vi "Parse VTG Sentence.vi"(8 "error in (no error)":errorcluster, 11 "VTG sentence":string) -> (0 "error out":errorcluster, 3 "VTG  data":T1 {"type of fix"."mode" items=["", "Simulator", "Not Valid", "Estimated", "Differential", "Autonomous"]})   [LabVIEW 2011, in "u-blox 5 Series.lvlib"]
doc: "Returns data contained in an NMEA sentence. You must manually select the polymorphic instance to use."
uses:
  u-blox 5 Series.lvlib
  typedefs/VTG Data.ctl
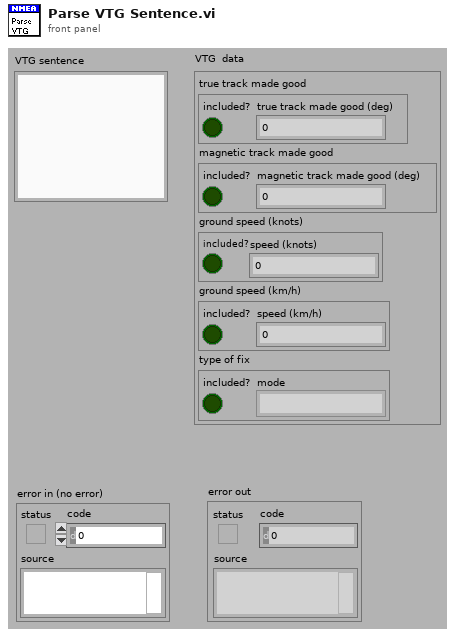
[diagram p1: front panel]
types:
  T1 = typedef "u-blox 5 Series.lvlib/VTG Data.ctl" = cluster{"true track made good":cluster{"included?":bool, "true track made good (deg)":dbl}, "magnetic track made good":cluster{"included?":bool, "magnetic track made good (deg)":dbl}, "ground speed (knots)":cluster{"included?":bool, "speed (knots)":dbl}, "ground speed (km/h)":cluster{"included?":bool, "speed (km/h)":dbl}, "type of fix":cluster{"included?":bool, "mode":u16}}
  T2 = cluster{"Boolean":bool, "True Track Made Good (Deg)":dbl}
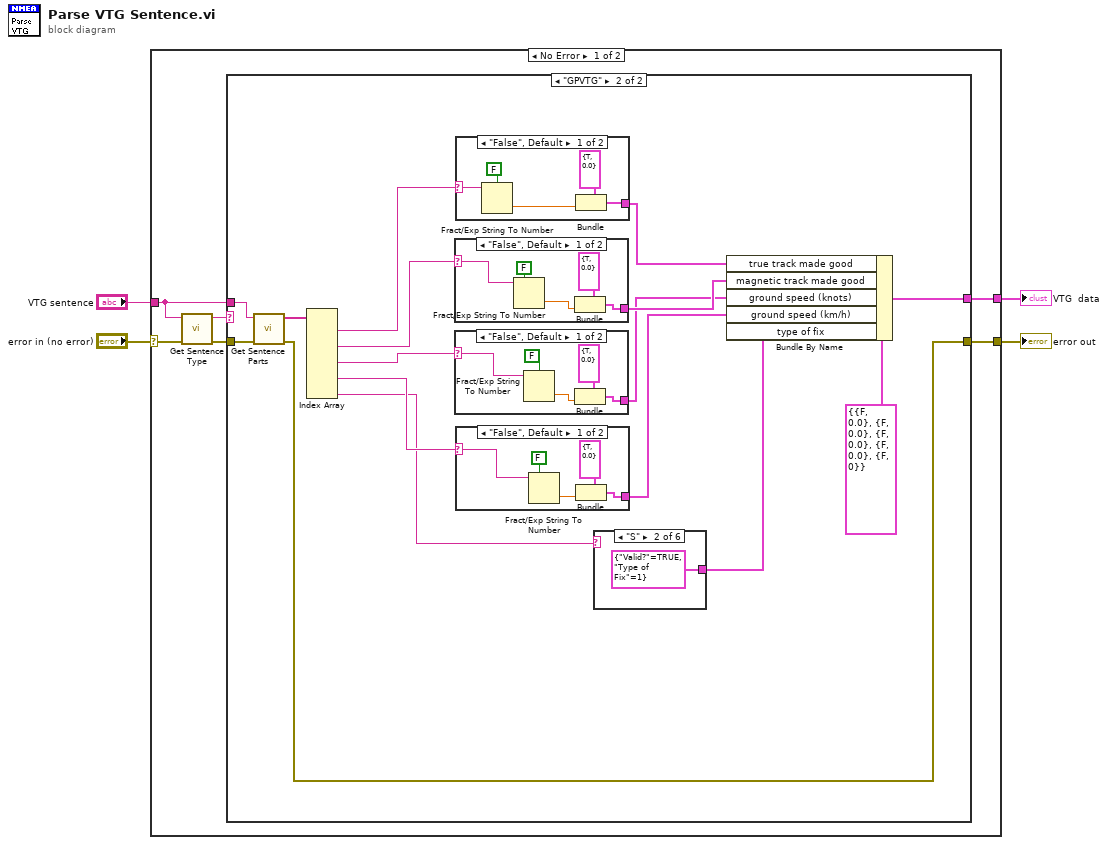
[diagram p0: block diagram]
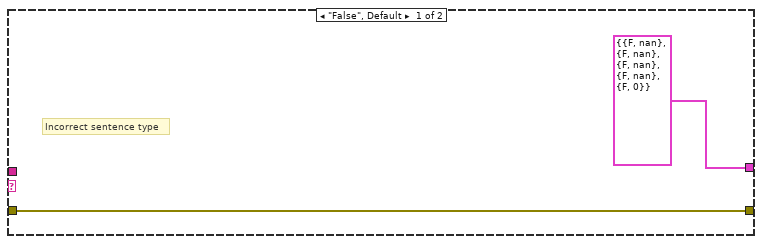
[diagram p2: hidden frame]
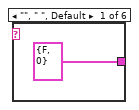
[diagram p3: hidden frame]
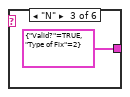
[diagram p4: hidden frame]
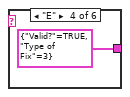
[diagram p5: hidden frame]
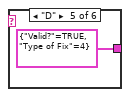
[diagram p6: hidden frame]
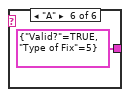
[diagram p7: hidden frame]
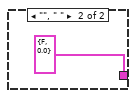
[diagram p8: hidden frame]
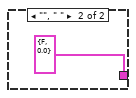
[diagram p9: hidden frame]
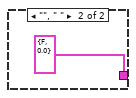
[diagram p10: hidden frame]
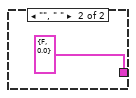
[diagram p11: hidden frame]
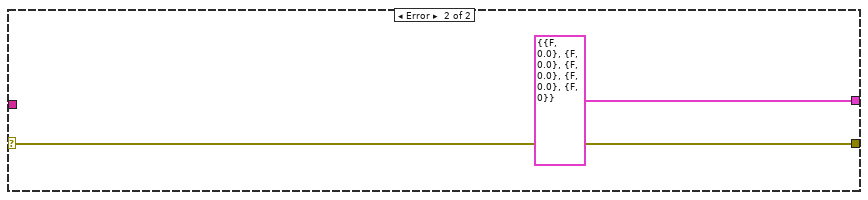
[diagram p12: hidden frame]
diagram:
  n1 = case shown="No Error" "error in (no error)" {
    selector: "error in (no error)" -> [w8 w59]
    tunnel: [w10 T1 {"true track made good"={"included?"=FALSE, "true track made good (deg)"=0.0}, "magnetic track made good"={"included?"=FALSE, "magnetic track made good (deg)"=0.0}, "ground speed (knots)"={"included?"=FALSE, "speed (knots)"=0.0}, "ground speed (km/h)"={"included?"=FALSE, "speed (km/h)"=0.0}, "type of fix"={"included?"=FALSE, "mode"=0}} ("VTG  Data")] -> w3
    tunnel: [w9 w59] -> w1
    tunnel: "VTG sentence" -> [w6 _]
    frame No Error {
      n2 = call "Get Sentence Type.vi"("error in (no error)"=w8, "sentence"=w6) -> ("error out"=w7:errorcluster, "sentence type"=w5:string)  [unwired: 2 in, 6 out]
      n3 = case shown="\"GPVTG\"" w5 {
        tunnel: w7 -> [w11 w28]
        tunnel: w6 -> [_ w15]
        tunnel: [T1 {"true track made good"={"included?"=FALSE, "true track made good (deg)"=nan}, "magnetic track made good"={"included?"=FALSE, "magnetic track made good (deg)"=nan}, "ground speed (knots)"={"included?"=FALSE, "speed (knots)"=nan}, "ground speed (km/h)"={"included?"=FALSE, "speed (km/h)"=nan}, "type of fix"={"included?"=FALSE, "mode"=0}} ("VTG  Data") w26] -> w10
        tunnel: [w11 w13] -> w9
        frame "False", Default {
          # "Incorrect sentence type"
        }
        frame "GPVTG" {
          n4 = call "Get Sentence Parts.vi"("error in (no error)"=w28, "sentence"=w15) -> ("error out"=w13:errorcluster, "sentence data"=w14:string[])  [unwired: 1 in, 7 out]
          n5 = Index Array(array=w14) -> (element #1=w24:string, element #3=w18:string, element #5=w19:string, element #7=w20:string, element #9=w17:string)  [unwired: 9 in, 4 out]
          n6 = case shown="\"False\", Default" w18 {
            selector: w18 -> [w48 _]
            tunnel: [w49 T2 {"Boolean"=FALSE, "True Track Made Good (Deg)"=0.0} ("True Track Made Good")] -> w23
            frame "False", Default {
              n7 = Fract/Exp String To Number(use system decimal point (T)=FALSE, string=w48) -> (number=w50:dbl)  [unwired: 3 out]
              n8 = Bundle(cluster=T2 {"Boolean"=TRUE, "True Track Made Good (Deg)"=0.0} ("True Track Made Good"), "True Track Made Good (Deg)"=w50) -> (w49:T2)  [unwired: 1 out]
            }
            frame "", " " {
            }
          }
          n9 = case shown="\"False\", Default" w19 {
            selector: w19 -> [w42 _]
            tunnel: [w43 T2 {"Boolean"=FALSE, "True Track Made Good (Deg)"=0.0} ("True Track Made Good")] -> w22
            frame "False", Default {
              n10 = Fract/Exp String To Number(use system decimal point (T)=FALSE, string=w42) -> (number=w44:dbl)  [unwired: 3 out]
              n11 = Bundle(cluster=T2 {"Boolean"=TRUE, "True Track Made Good (Deg)"=0.0} ("True Track Made Good"), "True Track Made Good (Deg)"=w44) -> (w43:T2)  [unwired: 1 out]
            }
            frame "", " " {
            }
          }
          n12 = case shown="\"False\", Default" w24 {
            selector: w24 -> [w54 _]
            tunnel: [w55 T2 {"Boolean"=FALSE, "True Track Made Good (Deg)"=0.0} ("True Track Made Good")] -> w25
            frame "False", Default {
              n13 = Fract/Exp String To Number(use system decimal point (T)=FALSE, string=w54) -> (number=w56:dbl)  [unwired: 3 out]
              n14 = Bundle(cluster=T2 {"Boolean"=TRUE, "True Track Made Good (Deg)"=0.0} ("True Track Made Good"), "True Track Made Good (Deg)"=w56) -> (w55:T2)  [unwired: 1 out]
            }
            frame "", " " {
            }
          }
          n15 = case shown="\"False\", Default" w20 {
            selector: w20 -> [w36 _]
            tunnel: [w37 T2 {"Boolean"=FALSE, "True Track Made Good (Deg)"=0.0} ("True Track Made Good")] -> w21
            frame "False", Default {
              n16 = Fract/Exp String To Number(use system decimal point (T)=FALSE, string=w36) -> (number=w38:dbl)  [unwired: 3 out]
              n17 = Bundle(cluster=T2 {"Boolean"=TRUE, "True Track Made Good (Deg)"=0.0} ("True Track Made Good"), "True Track Made Good (Deg)"=w38) -> (w37:T2)  [unwired: 1 out]
            }
            frame "", " " {
            }
          }
          n18 = case shown="\"S\"" w17 {
            tunnel: [cluster{"Valid?":bool, "Type of Fix":u16} {"Valid?"=FALSE, "Type of Fix"=0} ("Type of Fix") cluster{"Valid?":bool, "Type of Fix":u16} {"Valid?"=TRUE, "Type of Fix"=1} ("Type of Fix") cluster{"Valid?":bool, "Type of Fix":u16} {"Valid?"=TRUE, "Type of Fix"=2} ("Type of Fix") cluster{"Valid?":bool, "Type of Fix":u16} {"Valid?"=TRUE, "Type of Fix"=3} ("Type of Fix") cluster{"Valid?":bool, "Type of Fix":u16} {"Valid?"=TRUE, "Type of Fix"=4} ("Type of Fix") cluster{"Valid?":bool, "Type of Fix":u16} {"Valid?"=TRUE, "Type of Fix"=5} ("Type of Fix")] -> w16
            frame "", " ", Default {
            }
            frame "S" {
            }
            frame "N" {
            }
            frame "E" {
            }
            frame "D" {
            }
            frame "A" {
            }
          }
          n19 = Bundle By Name(cluster=T1 {"true track made good"={"included?"=FALSE, "true track made good (deg)"=0.0}, "magnetic track made good"={"included?"=FALSE, "magnetic track made good (deg)"=0.0}, "ground speed (knots)"={"included?"=FALSE, "speed (knots)"=0.0}, "ground speed (km/h)"={"included?"=FALSE, "speed (km/h)"=0.0}, "type of fix"={"included?"=FALSE, "mode"=0}} ("VTG  Data"), "true track made good"=w25, "magnetic track made good"=w23, "ground speed (knots)"=w22, "ground speed (km/h)"=w21, "type of fix"=w16) -> (w26:T1)
        }
      }
    }
    frame Error {
    }
  }
  "error out" <- w1
  "VTG  data" <- w3
